vi "SLL DE Decimate 2D Array.vi"(6 "Multi Time Stamp":timestamp[](array[timestamp]), 7 "Ref Array":sgl[][](array[numeric]), 8 "error in (no error)":errorcluster, 9 "Decimation Rate":i32, 10 "Mod":i32, 11 "Data Array":sgl[][](array[numeric])) -> (0 "error out":errorcluster, 1 "Time array":timestamp[](array[timestamp]), 2 "Mod Out":i32, 3 "Data Array Out":sgl[][](array[numeric]))   [LabVIEW 2009]
doc: "Copyright © 2005, Soliton Technologies.\nAll rights reserved."
panel:
  out "Array":i32[](array[numeric])
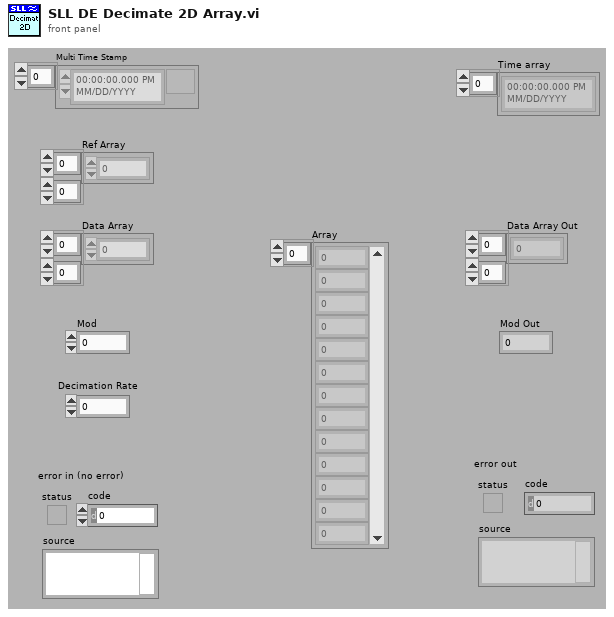
[diagram p1: front panel]
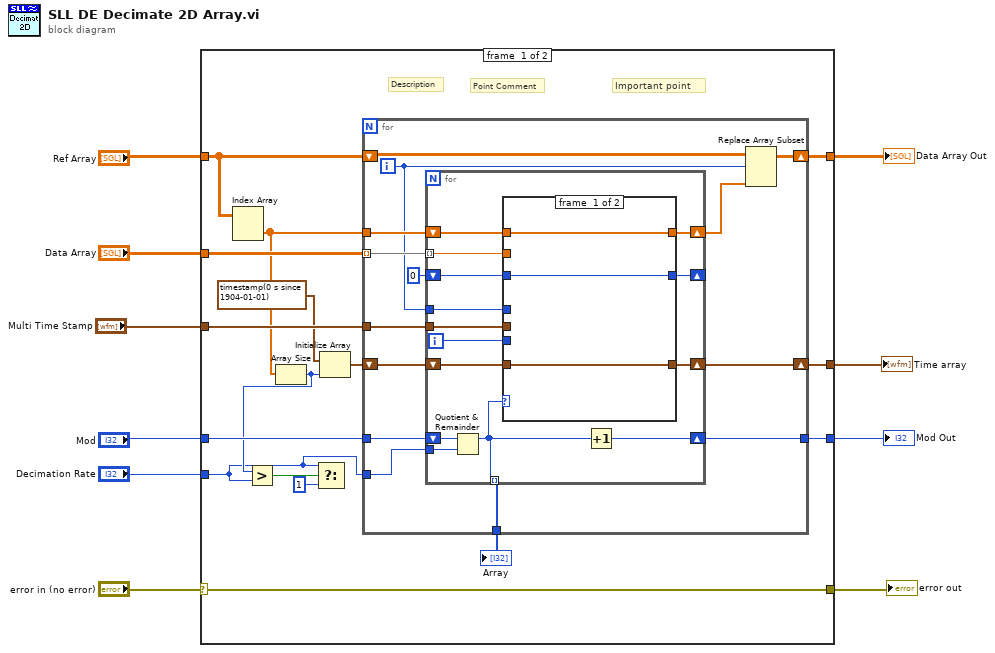
[diagram p0: block diagram]
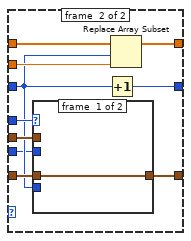
[diagram p2: hidden frame]
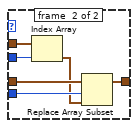
[diagram p3: hidden frame]
diagram:
  n1 = case shown="No Error" "error in (no error)" {
    selector: "error in (no error)" -> [w26 w78]
    tunnel: [w26 w78] -> w9
    tunnel: "Ref Array" -> [w25 _]
    tunnel: "Data Array" -> [w24 w77]
    tunnel: "Decimation Rate" -> [w11 _]
    tunnel: "Mod" -> [w17 w76]
    tunnel: [w23 w76] -> w4
    tunnel: [w13 w77] -> w1
    tunnel: "Multi Time Stamp" -> [w22 w75]
    tunnel: [w18 w75] -> w2
    frame #0 {
      # "Point Comment"
      # "Important point"
      # "Description"
      n2 = Index Array(array=w25) -> (element=w21:sgl[])  [unwired: 2 in]
      n3 = Array Size(array=w21) -> (size(s)=w16:i32)
      n4 = Greater?(x=w16, y=w11) -> (0:w15:bool)
      n5 = Select(t=w11, s=w15, f=1) -> ()  [unwired: 1 out]
      n6 = Initialize Array(timestamp(0 s since 1904-01-01), w16) -> (w19:timestamp[])
      n7 = for {
        tunnel: w24 -> [w36] mode=indexing
        tunnel: w11 -> [w39]
        tunnel: [w38] -> w23
        tunnel: w17 -> [w37]
        tunnel: w21 -> [w35]
        shift-right: [w33] -> w13
        shift-left: w25 -> [w34]
        tunnel: w22 -> [w31]
        shift-right: [w28] -> w18
        shift-left: w19 -> [w29]
        tunnel: [w27] -> w12
        i -> [w30]
        n8 = for {
          tunnel: w36 -> [w52] mode=indexing
          shift-right: [w53] -> w32
          shift-left: w35 -> [w54]
          shift-right: [w50] -> _
          shift-left: 0 -> [w51]
          tunnel: w39 -> [w49]
          shift-right: [w48] -> w38
          shift-left: w37 -> [w47]
          tunnel: w31 -> [w46]
          tunnel: w30 -> [w45]
          shift-right: [w44] -> w28
          shift-left: w29 -> [w43]
          tunnel: [w41] -> w27 mode=indexing
          i -> [w42]
          n9 = Quotient & Remainder(x=w47, y=w49) -> (x-y*floor(x/y)=w41:i32)  [unwired: 1 out]
          n10 = case shown="0" w41 {
            tunnel: w54 -> [w57 w67]
            tunnel: [w57 w66] -> w53
            tunnel: w52 -> [_ w65]
            tunnel: w51 -> [w56 w59]
            tunnel: [w56 w64] -> w50
            tunnel: w46 -> [_ w62]
            tunnel: w45 -> [_ w63]
            tunnel: [w55 w61] -> w44
            tunnel: w43 -> [w55 w60]
            tunnel: w42 -> [_ w58]
            frame #0 {
            }
            frame #1 {
              n11 = case shown="0" w63 {
                tunnel: w62 -> [_ w71]
                tunnel: [w68 w74] -> w61
                tunnel: w60 -> [w68 w73]
                tunnel: w59 -> [_ w72]
                tunnel: w58 -> [_ w69]
                frame #0 {
                }
                frame #1 {
                  n12 = Index Array(array=w71, index=w69) -> (element=w70:timestamp)
                  n13 = Replace Array Subset(array=w73, new element=w70, index=w72) -> (w74:timestamp[])
                }
              }
              n14 = Increment(x=w59) -> (x+1=w64:i32)
              n15 = Replace Array Subset(array=w67, new element=w65, index=w59) -> (w66:sgl[])
            }
          }
          n16 = Increment(x=w41) -> (x+1=w48:i32)
        }
        n17 = Replace Array Subset(array=w34, new element=w32, index (row)=w30) -> (w33:sgl[][])  [unwired: 1 in]
      }
      "Array" <- w12
    }
    frame #1 {
    }
  }
  "error out" <- w9
  "Mod Out" <- w4
  "Data Array Out" <- w1
  "Time array" <- w2
